vi "Error Code Converter.vi"(8 "error in (no error)":errorcluster, 9 "Error Code":i32, 10 "Additional Description":string, 11 "Potentiostat Galvanostat in":refnum<class "Potentiostat Galvanostat.lvclass">) -> (0 "error out":errorcluster, 3 "Potentiostat Galvanostat out":refnum<class "Potentiostat Galvanostat.lvclass">)   [LabVIEW 2018, in "Potentiostat Galvanostat.lvclass"]
uses:
  Potentiostat Galvanostat.lvclass
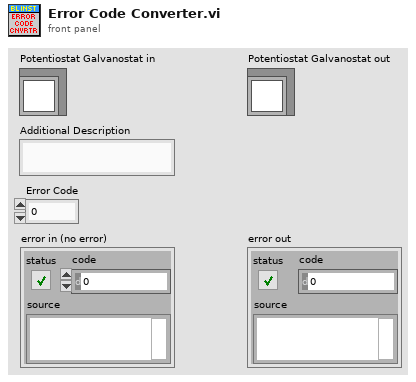
[diagram p1: front panel]
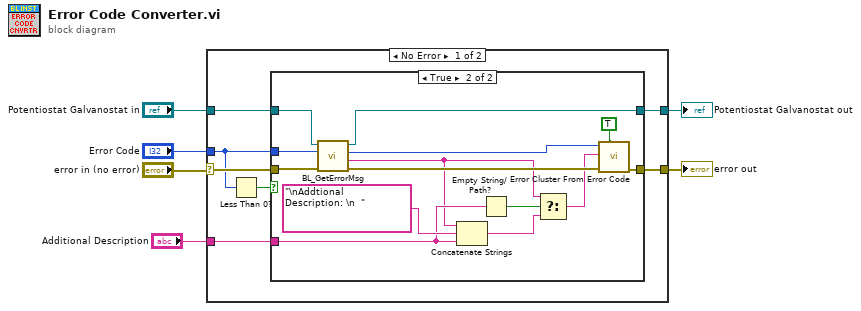
[diagram p0: block diagram]
diagram:
  n1 = case shown="No Error" "error in (no error)" {
    selector: "error in (no error)" -> [w12 w31]
    tunnel: [w10 w31] -> w6
    tunnel: "Error Code" -> [w11 _]
    tunnel: "Potentiostat Galvanostat in" -> [w9 w30]
    tunnel: [w8 w30] -> w2
    tunnel: "Additional Description" -> [w7 _]
    frame No Error {
      n2 = Less Than 0?(x=w11) -> (x < 0?=w13:bool)
      n3 = case shown="True" w13 {
        tunnel: w12 -> [w15 w23]
        tunnel: w11 -> [_ w22]
        tunnel: [w15 w29] -> w10
        tunnel: w9 -> [w14 w24]
        tunnel: [w14 w25] -> w8
        tunnel: w7 -> [_ w20]
        frame False {
        }
        frame True {
          n4 = call-dynamic "BL_GetErrorMsg.vi"("error in (no error)"=w23, "Error Code"=w22, "Potentiostat Galvanostat in"=w24) -> ("error out"=w27:errorcluster, "Error Message"=w17:string, "Error Code"=w26:i32, "Potentiostat Galvanostat out"=w25:refnum<class "Potentiostat Galvanostat.lvclass">)  [unwired: 5 in]
          n5 = Concatenate Strings(w17, "\nAddtional Description: \n  " ("string"), w20) -> (w19:string)
          n6 = Empty String/Path?(string/path=w20) -> (empty?=w16:bool)
          n7 = Select(t=w17, s=w16, f=w19) -> (s? t:f=w18:string)
          n8 = call <vilib>:"Error Cluster From Error Code.vi"("show call chain? (False)"=TRUE, "error in (no error)"=w27, "error message (\"\")"=w18, "error code (0)"=w26) -> ("error out"=w29:errorcluster)  [unwired: 5 in]
        }
      }
    }
    frame Error {
    }
  }
  "Potentiostat Galvanostat out" <- w2
  "error out" <- w6
